vi "getColorTemplate.vi"(8 "error in (no error)":errorcluster, 11 "Template Path":path=path "C:/Users/anton/Desktop/liquenes/lichen1.png") -> (0 "error out":errorcluster, 3 "Image Out":T1)   [LabVIEW 2018]
uses:
  <vilib>/vision/Image Controls.llb/IMAQ Image.ctl
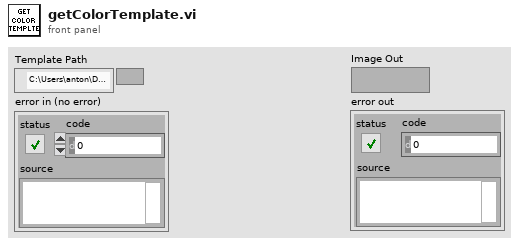
[diagram p1: front panel]
types:
  T1 = typedef "IMAQ Image.ctl" = refnum<image>
  T2 = typedef "Image Type" = u32
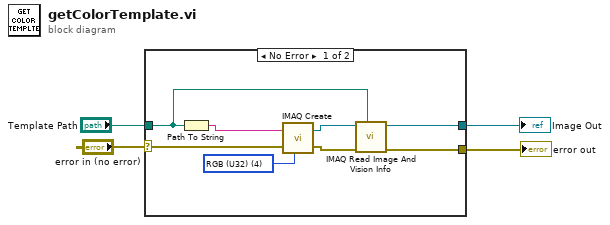
[diagram p0: block diagram]
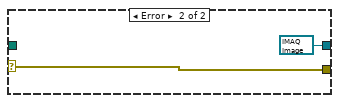
[diagram p2: hidden frame]
diagram:
  n1 = case shown="No Error" "error in (no error)" {
    selector: "error in (no error)" -> [w11 w13]
    tunnel: "Template Path" -> [w7 _]
    tunnel: [w6 w13] -> w1
    tunnel: [w5 T1 refnum ("Image Out")] -> w2
    frame No Error {
      w10 = T2 4 items=["Grayscale (U8)", "Grayscale (I16)", "Grayscale (SGL)", "Complex (CSG)", "RGB (U32)", "HSL (U32)", "RGB (U64)", "Grayscale (U16)"] ("Image Type")
      n2 = Path To String(path=w7) -> (string=w12:string)
      n3 = call "IMAQ Create"("Image Name"=w12, "Image Type"=w10, "error in (no error)"=w11) -> ("New Image"=w9:T1, "error out"=w8:errorcluster)  [unwired: 1 in, 1 out]
      n4 = call "IMAQ Read Image And Vision Info"("File Path"=w7, "error in (no error)"=w8, "Image"=w9) -> ("error out"=w6:errorcluster, "Image Out"=w5:T1)  [unwired: 1 in, 6 out]
    }
    frame Error {
    }
  }
  "Image Out" <- w2
  "error out" <- w1
